vi "test Connect Disconnect.vi"(8 "error in (no error)":errorcluster, 11 "TestCase in":refnum<class "SLSC Switch Messaging Tests.lvclass">) -> (0 "error out":errorcluster, 3 "TestCase out":refnum<class "SLSC Switch Messaging Tests.lvclass">)   [LabVIEW 2017, in "SLSC Switch Messaging Tests.lvclass"]
uses:
  SLSC Switch Messaging Tests.lvclass
  Includes/CDMessaging.lvlibp/Switch/Switch Disconnect Message/Switch Disconnect Message.lvclass
  C:/Dev/GitHub/niveristand-slsc-switch-message-library/Includes/CDMessaging.lvlibp/Message/Abstract Message/Abstract Message.lvclass
  Includes/CDMessaging.lvlibp/Switch/Switch Connect Message/Switch Connect Message.lvclass
  Support/Mock SLSC Switch Consumer.lvclass
  SLSC Switch Messaging Tests.lvclass/SLSC Switch Messaging Tests.ctl
  Support/Mock SLSC Switch Consumer.lvclass/Mock SLSC Switch Consumer.ctl
  Support/Read Connections.vi
  Includes/CDMessaging.lvlibp/Switch/Abstract Switch Consumer/Abstract Switch Consumer.lvclass
  C:/Dev/GitHub/niveristand-slsc-switch-message-library/Includes/CDMessaging.lvlibp/Consumer/Abstract Consumer/Abstract Consumer.lvclass
  Includes/CDMessaging.lvlibp/Producer/Abstract Producer/Abstract Producer.lvclass
  <vilib>/addons/_JKI Toolkits/VI Tester/TestCase.llb/TestCase.lvclass
  Includes/CDMessaging.lvlibp/Consumer/Abstract Consumer/Abstract Consumer.lvclass
  C:/Program Files (x86)/National Instruments/LabVIEW 2017/vi.lib/addons/_JKI Toolkits/VI Tester/TestCase.llb/TestCase.lvclass
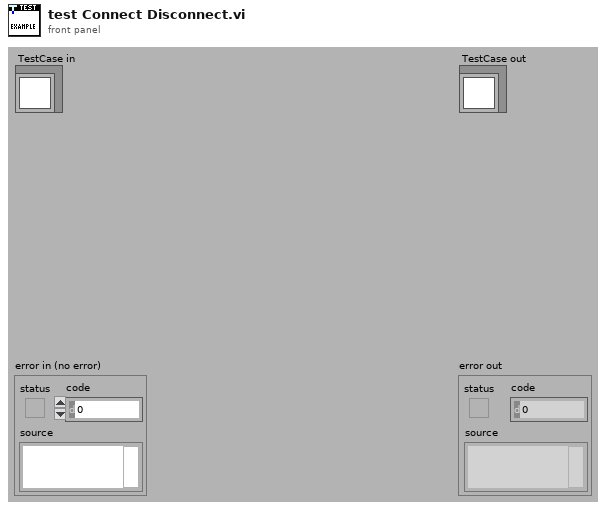
[diagram p1: front panel]
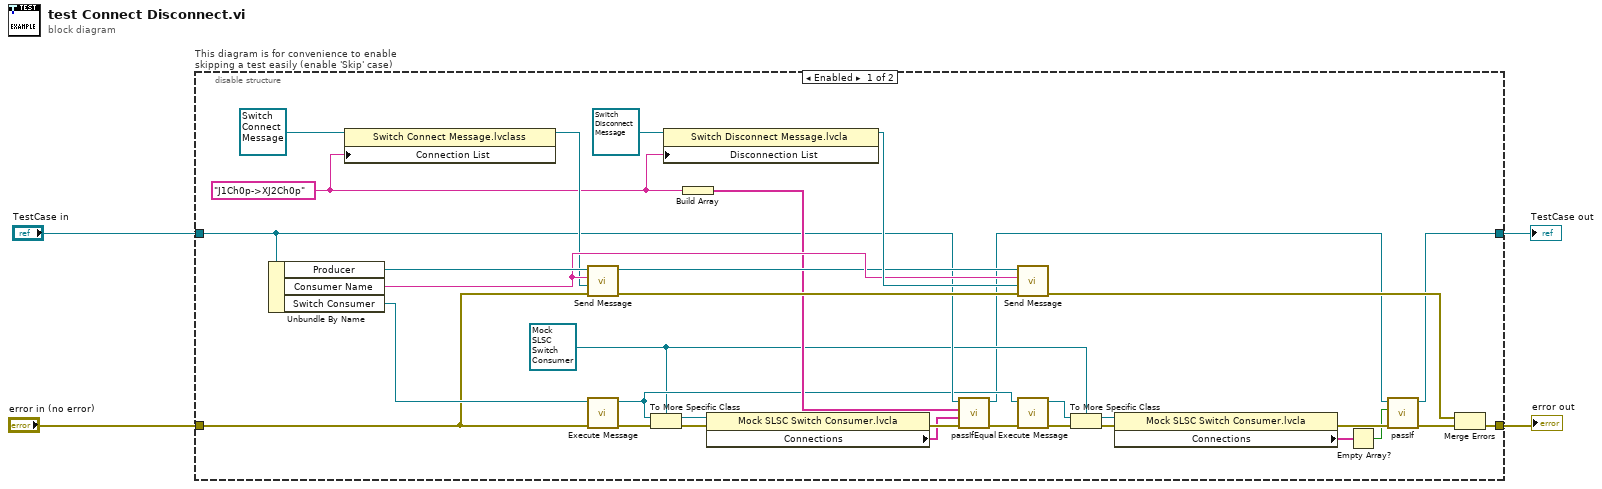
[diagram p0: block diagram]
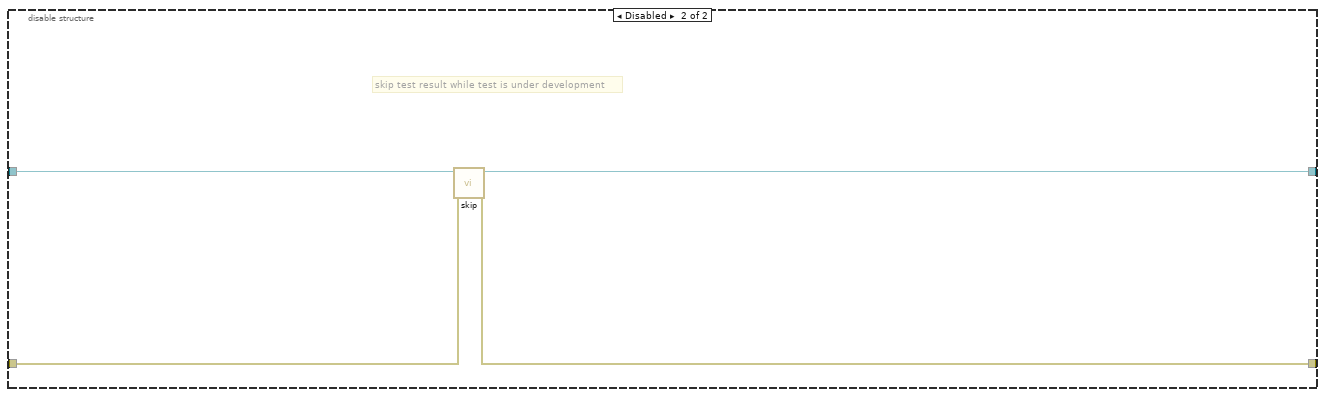
[diagram p2: hidden frame]
diagram:
  n1 = disable-structure "This diagram is for convenience to enable skipping a test easily (enable 'Skip' case)" shown="Enabled" {
    disable-tunnel: "TestCase in" -> [w17 w41]
    disable-tunnel: [w8 w39] -> w1
    disable-tunnel: [w33 w40] -> w3
    disable-tunnel: "error in (no error)" -> [w30 w38]
    frame Enabled {
      w12 = refnum<class "Mock SLSC Switch Consumer.lvclass"> refnum ("Mock SLSC Switch Consumer.lvclass")
      w20 = "J1Ch0p->XJ2Ch0p"
      n2 = Unbundle By Name(w17) -> ("Producer"=w32:refnum<class "Abstract Producer.lvclass">, "Consumer Name"=w31:string, "Switch Consumer"=w35:refnum<class "Abstract Switch Consumer.lvclass">)
      n3 = property class="Switch Connect Message.lvclass"(reference=refnum<class "Switch Connect Message.lvclass"> refnum ("CDMessaging.lvlibp:Switch Connect Message.lvclass"), "Connection List"=w20) -> (reference out=w26:refnum<class "Switch Connect Message.lvclass">)  [unwired: 1 in, 1 out]
      n4 = call-dynamic "Send Message.vi"("error in (no error)"=w30, "Message in"=w26, "Consumer in"=w31, "Abstract Producer in"=w32) -> ("error out"=w29:errorcluster, "Abstract Producer out"=w28:refnum<class "Abstract Producer.lvclass">)  [unwired: 4 in, 2 out]
      n5 = call "Execute Message.vi"("error in (no error)"=w30, "Abstract Consumer in"=w35) -> ("error out"=w25:errorcluster, "Abstract Consumer out"=w16:refnum<class "Abstract Consumer.lvclass">)  [unwired: 6 in, 2 out]
      n6 = To More Specific Class(target class=w12, reference=w16, error in=w25) -> (specific class reference=w23:refnum<class "Mock SLSC Switch Consumer.lvclass">, error out=w24:errorcluster)
      n7 = property class="Switch Disconnect Message.lvcla"(reference=refnum<class "Switch Disconnect Message.lvclass"> refnum ("CDMessaging.lvlibp:Switch Disconnect Message.lvclass"), "Disconnection List"=w20) -> (reference out=w36:refnum<class "Switch Disconnect Message.lvclass">)  [unwired: 1 in, 1 out]
      n8 = Build Array(w20) -> (w19:string[])
      n9 = property class="Mock SLSC Switch Consumer.lvcla"(reference=w23, error in=w24) -> (error out=w22:errorcluster, "Connections"=w21:string[])  [unwired: 1 out]
      n10 = call-dynamic "passIfEqual.vi"("error in (no error)"=w22, "y"=w21, "x"=w19, "TestCase in"=w17) -> ("error out"=w18:errorcluster, "TestCase out"=w9:refnum<class "SLSC Switch Messaging Tests.lvclass">)  [unwired: 6 in]
      n11 = call-dynamic "Send Message.vi"("error in (no error)"=w29, "Message in"=w36, "Consumer in"=w31, "Abstract Producer in"=w28) -> ("error out"=w34:errorcluster)  [unwired: 4 in, 3 out]
      n12 = call "Execute Message.vi"("error in (no error)"=w18, "Abstract Consumer in"=w16) -> ("error out"=w14:errorcluster, "Abstract Consumer out"=w13:refnum<class "Abstract Consumer.lvclass">)  [unwired: 6 in, 2 out]
      n13 = To More Specific Class(target class=w12, reference=w13, error in=w14) -> (specific class reference=w7:refnum<class "Mock SLSC Switch Consumer.lvclass">, error out=w15:errorcluster)
      n14 = property class="Mock SLSC Switch Consumer.lvcla"(reference=w7, error in=w15) -> (error out=w11:errorcluster, "Connections"=w6:string[])  [unwired: 1 out]
      n15 = Empty Array?(array=w6) -> (empty?=w5:bool)
      n16 = call-dynamic "passIf.vi"("error in (no error)"=w11, "pass"=w5, "TestCase in"=w9) -> ("error out"=w10:errorcluster, "TestCase out"=w8:refnum<class "SLSC Switch Messaging Tests.lvclass">)  [unwired: 7 in]
      n17 = Merge Errors(w34, w10) -> (w33:errorcluster)
    }
    frame Disabled {
      # "skip test result while test is under development"
      n18 = call <vilib>:"skip.vi"("error in (no error)"=w38, "TestCase in"=w41) -> ("error out"=w40:errorcluster, "TestCase out"=w39:refnum<class "SLSC Switch Messaging Tests.lvclass">)  [unwired: 8 in]
    }
  }
  "error out" <- w3
  "TestCase out" <- w1
